vi "calculate d phase.vi"(6 "threshold":dbl=50.0 format="%0.2f", 9 "IQ in":cdb[][](array[numeric]), 10 "dt":dbl, 11 "center frequency (Hz)":dbl) -> (1 "d amp":dbl[][](array[numeric]), 2 "amp":dbl[](array[numeric]), 3 "spectrum":cluster{"f0":dbl, "df":dbl, "magnitude":dbl[]}[](array[cluster]), 4 "d phase":dbl[][](array[numeric]), 5 "frequncy":dbl[](array[numeric]))   [LabVIEW 2021]
uses:
  <vilib>/Analysis/4window.llb/windowTd.ctl
  <vilib>/Analysis/coordinate.llb/Angle Units.ctl
  <vilib>/Analysis/coordinate.llb/Angle Range (Degree).ctl
  <vilib>/Analysis/coordinate.llb/Wrap Angle (scalar).vi
  <vilib>/measure/maspectr.llb/FFT Spectrum (Mag-Phase) for 1 Chan (CDB).vi
  <vilib>/Analysis/NI_AALPro.lvlib
  <vilib>/measure/NI_MAPro.lvlib
  <vilib>/Analysis/NI_AAL_SigProc.lvlib
  <vilib>/Analysis/NI_AAL_Angle.lvlib
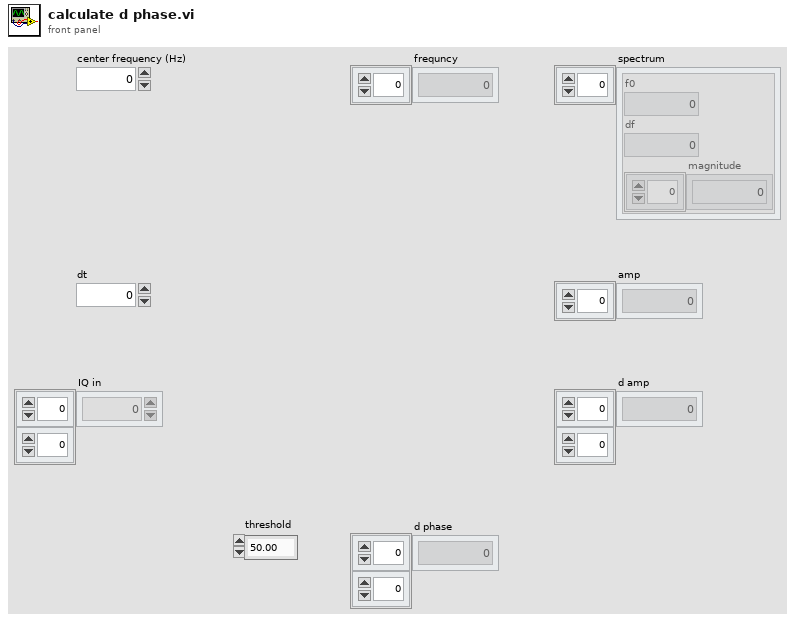
[diagram p1: front panel]
types:
  T1 = cluster{"dB On (F)":bool, "unwrap phase (F)":bool, "convert to degree (F)":bool}
  T2 = typedef "NI_AALPro.lvlib/windowTd.ctl" = u32
  T3 = typedef "NI_AAL_Angle.lvlib/Angle Range (Degree).ctl" = u16
  T4 = typedef "NI_AAL_Angle.lvlib/Angle Units.ctl" = i32
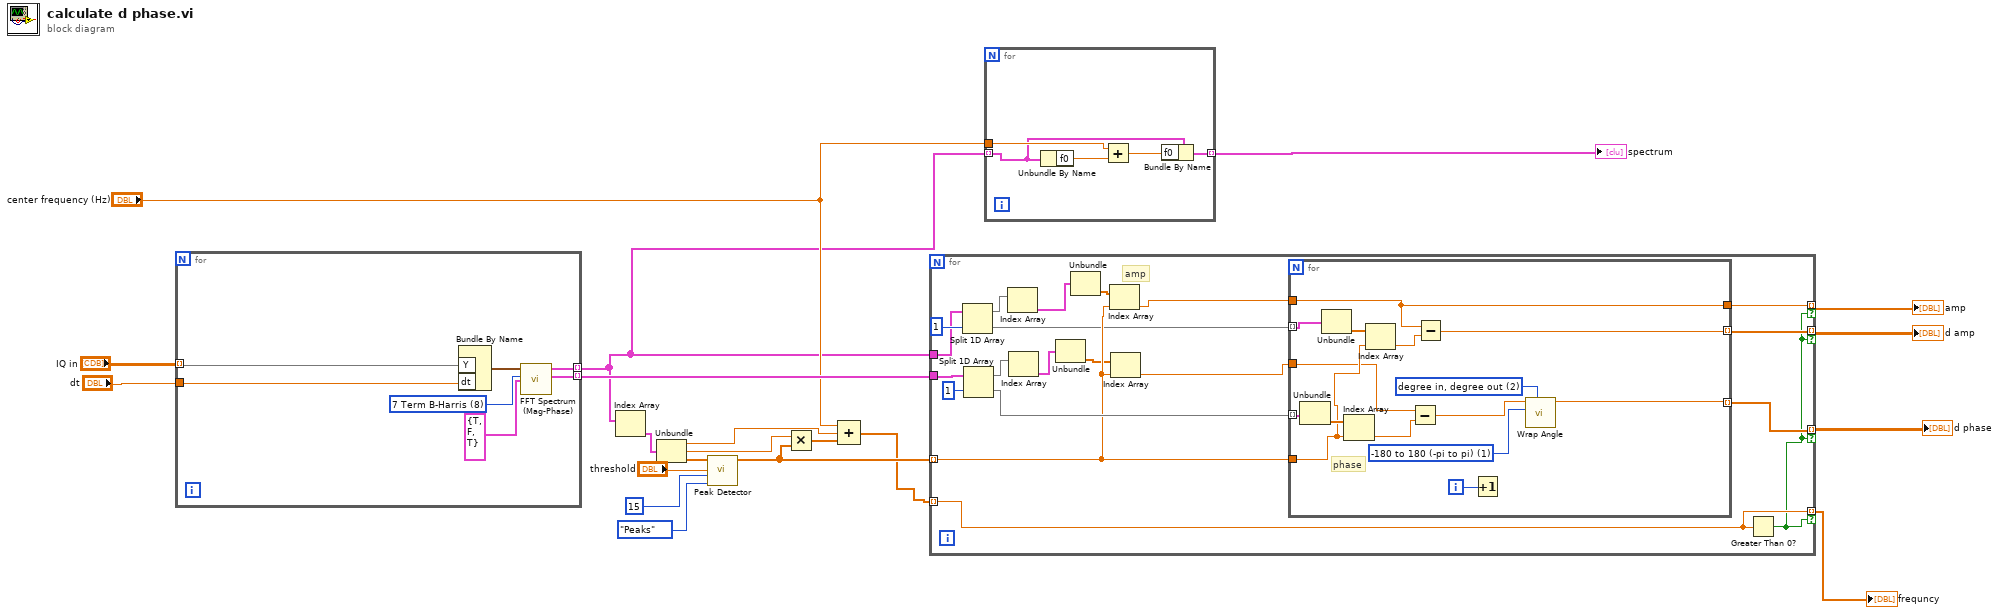
[diagram p0: block diagram]
diagram:
  n1 = for {
    tunnel: "dt" -> [w25]
    tunnel: [w23] -> w4 mode=indexing
    tunnel: [w22] -> w12 mode=indexing
    tunnel: "IQ in" -> [w21] mode=indexing
    w26 = T2 8 items=["Rectangle"=0, "Hanning"=1, "Hamming"=2, "Blackman-Harris"=3, "Exact Blackman"=4, "Blackman"=5, "Flat Top"=6, "4 Term B-Harris "=7, "7 Term B-Harris"=8, "Low Sidelobe"=9, "Blackman Nuttall"=11, "Triangle"=30, "Bartlett-Hanning"=31, "Bohman"=32, "Parzen"=33, "Welch"=34, "Kaiser"=60, "Dolph-Chebyshev"=61, "Gaussian"=62] ("window")
    n2 = Bundle By Name("Y"=w21, "dt"=w25) -> (w27:waveform(cdb))  [unwired: 1 in]
    n3 = call-poly <vilib>:"FFT Spectrum (Mag-Phase).vi"("view"=T1 {"dB On (F)"=TRUE, "unwrap phase (F)"=FALSE, "convert to degree (F)"=TRUE}, "window"=w26, "time signal"=w27) -> ("phase"=w22:cluster{"f0":dbl, "df":dbl, "phase":dbl[]}, "magnitude"=w23:cluster{"f0":dbl, "df":dbl, "magnitude":dbl[]})  [unwired: 4 in, 3 out]
  }
  n4 = Index Array(array=w4) -> (element=w7:cluster{"f0":dbl, "df":dbl, "magnitude":dbl[]})  [unwired: 1 in]
  n5 = Unbundle(w7) -> ("f0"=w16:dbl, "df"=w14:dbl, "magnitude"=w8:dbl[])
  n6 = call <vilib>:"Peak Detector.vi"("peaks/valleys"=enum32{"Peaks", "Valleys"}."Peaks", "width"=15, "threshold"="threshold", "X"=w8) -> ("Locations"=w13:dbl[])  [unwired: 3 in, 4 out]
  n7 = Multiply(x=w14, y=w13) -> (x*y=w15:dbl[])
  n8 = Compound Arithmetic op=ADD("center frequency (Hz)", w16, w15) -> (w2:dbl[])
  n9 = for {
    tunnel: w12 -> [w47]
    tunnel: w4 -> [w40]
    tunnel: w13 -> [w43] mode=indexing
    tunnel: [w32] -> w19 mode=indexing if=w28
    tunnel: [w31] -> w18 mode=indexing if=w28
    tunnel: [w30] -> w20 mode=indexing if=w28
    tunnel: w2 -> [w29] mode=indexing
    tunnel: [w29] -> w1 mode=indexing if=w28
    # "amp"
    n10 = Split 1D Array(array=w40, index=1) -> (first subarray=w42:cluster{"f0":dbl, "df":dbl, "magnitude":dbl[]}[], second subarray=w39:cluster{"f0":dbl, "df":dbl, "magnitude":dbl[]}[])
    n11 = Split 1D Array(array=w47, index=1) -> (first subarray=w45:cluster{"f0":dbl, "df":dbl, "phase":dbl[]}[], second subarray=w44:cluster{"f0":dbl, "df":dbl, "phase":dbl[]}[])
    n12 = Index Array(array=w42) -> (element=w37:cluster{"f0":dbl, "df":dbl, "magnitude":dbl[]})  [unwired: 1 in]
    n13 = Index Array(array=w45) -> (element=w35:cluster{"f0":dbl, "df":dbl, "phase":dbl[]})  [unwired: 1 in]
    n14 = Unbundle(w35) -> ("phase"=w36:dbl[])  [unwired: 2 out]
    n15 = Unbundle(w37) -> ("magnitude"=w38:dbl[])  [unwired: 2 out]
    n16 = Index Array(array=w38, index=w43) -> (element=w33:dbl)
    n17 = Index Array(array=w36, index=w43) -> (element=w34:dbl)
    n18 = for {
      tunnel: w44 -> [w61] mode=indexing
      tunnel: w43 -> [w58]
      tunnel: w39 -> [w59] mode=indexing
      tunnel: [w56] -> w32 mode=indexing
      tunnel: w33 -> [w48]
      tunnel: w34 -> [w51]
      tunnel: [w49] -> w31 mode=indexing
      tunnel: [w48] -> w30
      i -> [w50]
      w52 = T3 1 items=["none", "-180 to 180 (-pi to pi)", "0 to 360 (0 to 2pi)"] ("angle range")
      w54 = T4 2 items=["radian in, radian out", "radian in, degree out", "degree in, degree out", "degree in, radian out"] ("angle units")
      # "phase"
      n19 = Unbundle(w61) -> ("phase"=w62:dbl[])  [unwired: 2 out]
      n20 = Unbundle(w59) -> ("magnitude"=w60:dbl[])  [unwired: 2 out]
      n21 = Index Array(array=w62, index=w58) -> (element=w55:dbl)
      n22 = Index Array(array=w60, index=w58) -> (element=w57:dbl)
      n23 = Subtract(x=w51, y=w55) -> (x-y=w53:dbl)
      n24 = Subtract(x=w48, y=w57) -> (x-y=w56:dbl)
      n25 = Increment(x=w50) -> ()  [unwired: 1 out]
      n26 = call-poly <vilib>:"Wrap Angle.vi"("angle units"=w54, "angle range"=w52, "angle in"=w53) -> ("angle out"=w49:dbl)  [unwired: 7 in, 1 out]
    }
    n27 = Greater Than 0?(x=w29) -> (x > 0?=w28:bool)
  }
  "amp" <- w20
  "d amp" <- w19
  "d phase" <- w18
  "frequncy" <- w1
  n28 = for {
    tunnel: w4 -> [w65] mode=indexing
    tunnel: "center frequency (Hz)" -> [w66]
    tunnel: [w63] -> w3 mode=indexing
    n29 = Unbundle By Name(w65) -> ("f0"=w67:dbl)
    n30 = Add(x=w66, y=w67) -> (x+y=w64:dbl)
    n31 = Bundle By Name(cluster=w65, "f0"=w64) -> (w63:cluster{"f0":dbl, "df":dbl, "magnitude":dbl[]})
  }
  "spectrum" <- w3
